vi "APSxAddSensorASIC.vi"(8 "error in (no error)":errorcluster caption="错误输入（无错误）", 10 "hASIC":i32, 11 "hSENSOR":i32) -> (0 "error out":errorcluster caption="错误输出", 1 "hASIC out":i32, 2 "hSENSOR out":i32, 3 "Message":string)   [LabVIEW 2018]
doc: "该模板用于创建子VI。"
uses:
  APSx.dll/APSx.dll
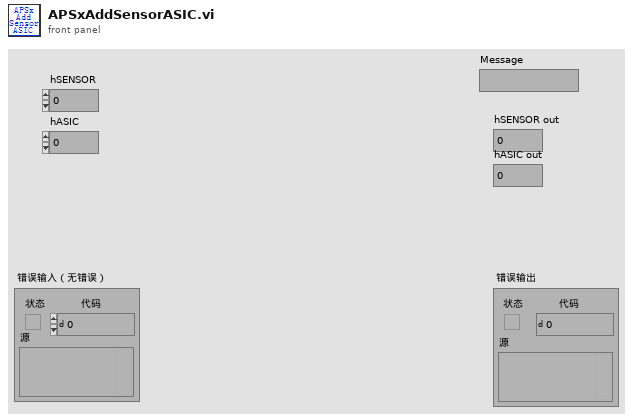
[diagram p1: front panel]
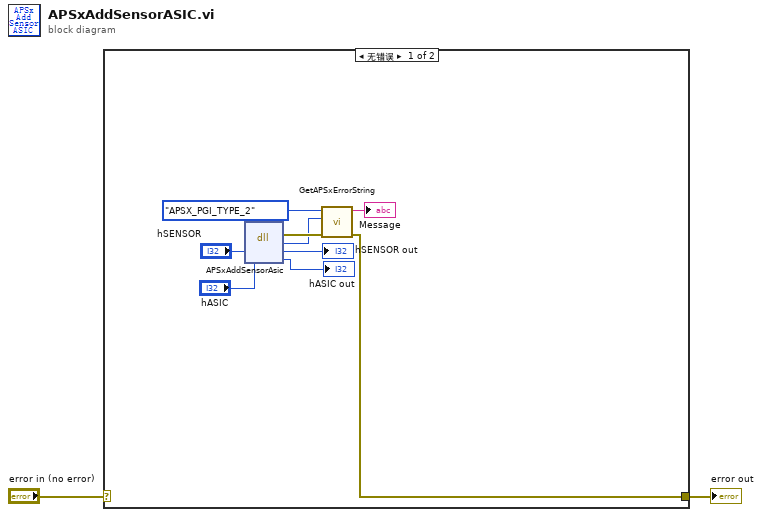
[diagram p0: block diagram]
diagram:
  n1 = case shown="无错误" "error in (no error)" {
    selector: "error in (no error)" -> [_ w12]
    tunnel: [w6 w12] -> w1
    frame No Error {
      n2 = dll-call lib="PTH2]abs D项目Feng恒隆项目Labview传感器对中台SourcesAPSx.dllAPSx.dll" fn="APSxAddSensorAsic"("hSENSOR"="hSENSOR", "hASIC"="hASIC") -> (error out=w9:errorcluster, "Code"=w8:i32, "hSENSOR"=→"hSENSOR out":i32, "hASIC"=→"hASIC out":i32)  [unwired: 3 in, 1 out]
      n3 = call "GetAPSxErrorString.vi"("error in (no error)"=w9, "ErrorCode"=w8, "PGIType"=enum16{"APSX_PGI_TYPE_1", "APSX_PGI_TYPE_2"}."APSX_PGI_TYPE_2") -> ("error out"=w6:errorcluster, "Message"=→"Message":string)  [unwired: 7 in]
    }
    frame Error {
    }
  }
  "error out" <- w1
